vi "Finish.vi"   [LabVIEW 2017]
doc: "This VI is called during exit. It can be used to close I/O refnums, save collected data, etc."
uses:
  <vilib>/Rock Robotics/WPI/Utilities/WPI_GetSetVariantRefNum.vi
types:
  T1 = typedef "WPI_JoystickDevRef.ctl" = cluster{"Device":T2}
  T2 = typedef "WPI_JoystickDeviceEnum.ctl" = enum16{"USB 0", "USB 1", "USB 2", "USB 3", "USB 4", "USB 5"}
  T3 = typedef "WPI_GyroDevRef.ctl" = cluster{"DevStatus":errorcluster, "Analog Channel":T4, "Gain (VoltsPerDegree/Second)":dbl, "Gyro Type":enum16{"Analog", "XRS450"}, "Handle":i32, "SPI Bus":T5, "Device Found":bool, "Sample Rate":dbl, "Calibrate On Open":bool, "Offset":dbl}
  T4 = typedef "FPGA_AIChannel.ctl" = enum8{"AI 0", "AI 1", "AI 2", "AI 3", "AI MXP 0", "AI MXP 1", "AI MXP 2", "AI MXP 3", "Invalid"}
  T5 = typedef "spi_bus.ctl" = enum16{"SPI On-Board, CS0", "SPI On-Board, CS1", "SPI On-Board, CS2", "SPI On-Board, CS3", "SPI MXP", "Invalid"}
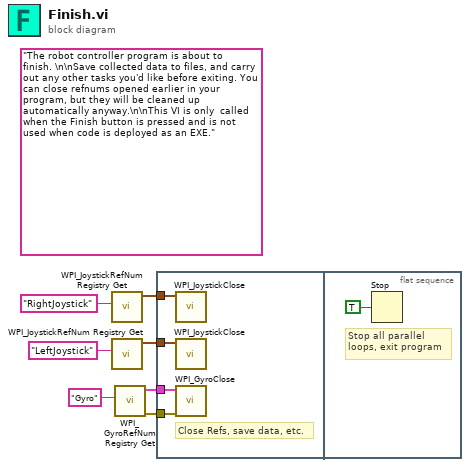
[diagram p0: block diagram]
diagram:
  (unwired) "The robot controller program is about to finish. \n\nSave collected data to files, and carry out any other tasks you'd like before exiting. You can close refnums opened earlier in your program, but they will be cleaned up automatically anyway.\n\nThis VI is only  called when the Finish button is pressed and is not used when code is deployed as an EXE."
  n1 = call <vilib>:"WPI_JoystickRefNum Registry Get.vi"("refnum name"="RightJoystick") -> ("JoystickDevRef"=w4:T1)  [unwired: 1 in, 9 out]
  n2 = call <vilib>:"WPI_JoystickRefNum Registry Get.vi"("refnum name"="LeftJoystick") -> ("JoystickDevRef"=w6:T1)  [unwired: 1 in, 9 out]
  n3 = call <vilib>:"WPI_GyroRefNum Registry Get.vi"("refnum name"="Gyro") -> ("error out"=w2:errorcluster, "GyroDevRef"=w1:T3)  [unwired: 9 in]
  n4 = flat-sequence {
    tunnel: w6 -> [w11]
    tunnel: w4 -> [w10]
    tunnel: w2 -> [w9]
    tunnel: w1 -> [w8]
    frame #0 {
      # "Close Refs, save data, etc."
      n5 = call <vilib>:"WPI_JoystickClose.vi"("JoystickDevRef"=w10) -> ()  [unwired: 11 out]
      n6 = call <vilib>:"WPI_JoystickClose.vi"("JoystickDevRef"=w11) -> ()  [unwired: 11 out]
      n7 = call <vilib>:"WPI_GyroClose.vi"("error in"=w9, "GyroDevRef"=w8) -> ()  [unwired: 9 in, 1 out]
    }
    frame #1 {
      # "Stop all parallel\nloops, exit program"
      n8 = Stop(stop? (T)=TRUE ("Quit")) -> ()
    }
  }
